vi "ComputeEandU (SubVI).vi"(11 "weights in":sgl[][](array[numeric])) -> (2 "e":sgl[](array[numeric]), 3 "u":sgl[](array[numeric]))   [LabVIEW 2011]
panel:
  out "final u":sgl
  out "final e":sgl
  out "Waveform Graph":sgl[][](graph)
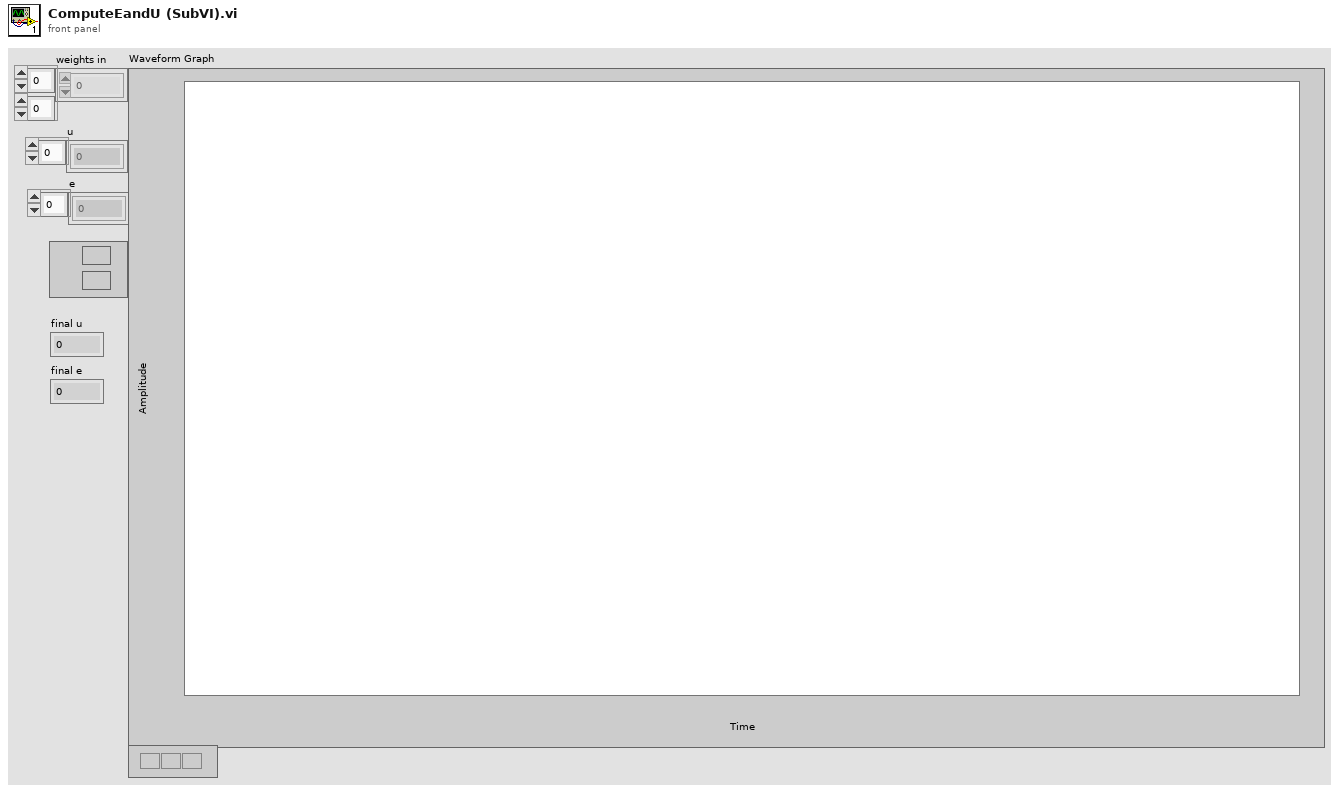
[diagram p1: front panel]
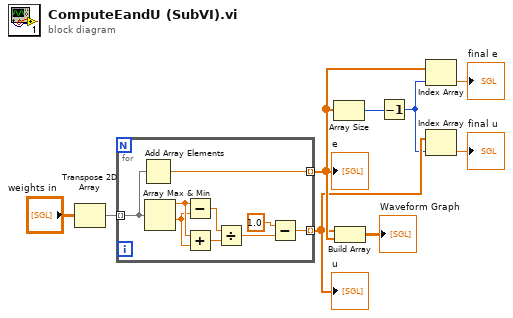
[diagram p0: block diagram]
diagram:
  n1 = Transpose 2D Array(2D array="weights in") -> (transposed array=w7:sgl[][])
  n2 = for {
    tunnel: w7 -> [w18] mode=indexing
    tunnel: [w17] -> w6 mode=indexing
    tunnel: [w10] -> w4 mode=indexing
    n3 = Add Array Elements(numeric array=w18) -> (sum=w17:sgl)
    n4 = Array Max & Min(array=w18) -> (max value=w15:sgl, min value=w14:sgl)  [unwired: 2 out]
    n5 = Subtract(x=w15, y=w14) -> (x-y=w16:sgl)
    n6 = Add(x=w15, y=w14) -> (x+y=w13:sgl)
    n7 = Divide(x=w16, y=w13) -> (x/y=w12:sgl)
    n8 = Subtract(x=sgl 1.0, y=w12) -> (x-y=w10:sgl)
  }
  "u" <- w4
  "e" <- w6
  n9 = Array Size(array=w6) -> (size(s)=w3:i32)
  n10 = Build Array(w4, w6) -> (→"Waveform Graph":sgl[][])
  n11 = Decrement(x=w3) -> (x-1=w1:i32)
  n12 = Index Array(array=w6, index=w1) -> (element=→"final e":sgl)
  n13 = Index Array(array=w4, index=w1) -> (element=→"final u":sgl)
